vi "AOTF Messenger.vi"(0 "AOTF Notifier Name":string, 2 "AOTF Action":T1, 5 "Wavelength (nm)":string, 7 "Power (%)":dbl, 9 "Line On/Off":bool, 11 "Beam Blank":bool) -> (4 "AOTF Notifier Name (Dup)":string, 6 "Wavelength (nm) Out":string, 8 "Power (%) Out":dbl, 10 "Line On/Off Out":bool, 13 "Wavelengths (nm)":string[](array[string]), 15 "Beam Blank Out":bool)   [LabVIEW 2016]
uses:
  AOTF Controls/AOTF Actions.ctl
  AOTF Controls/AOTF Notifier Element.ctl
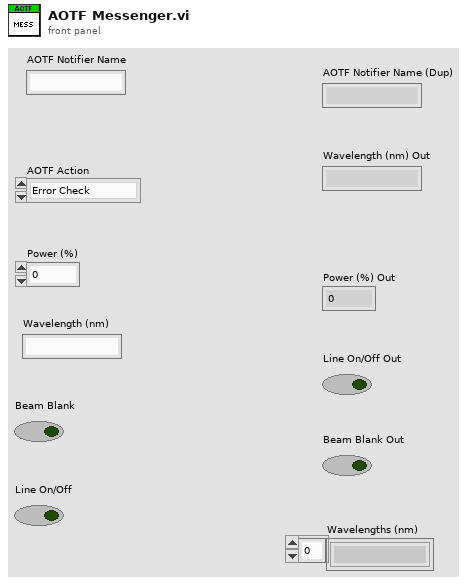
[diagram p1: front panel]
types:
  T1 = typedef "AOTF Actions.ctl" = enum16{"Error Check", "Blank", "Line On/Off", "Set Power", "Status", "Quit"}
  T2 = typedef "AOTF Notifier Element.ctl" = cluster{"AOTF Action":T1, "Laser Line":string, "Power (%)":dbl, "Beam Blank On/Off":bool, "Line On/Off":bool, "Error":errorcluster, "Wavelengths (nm)":string[]}
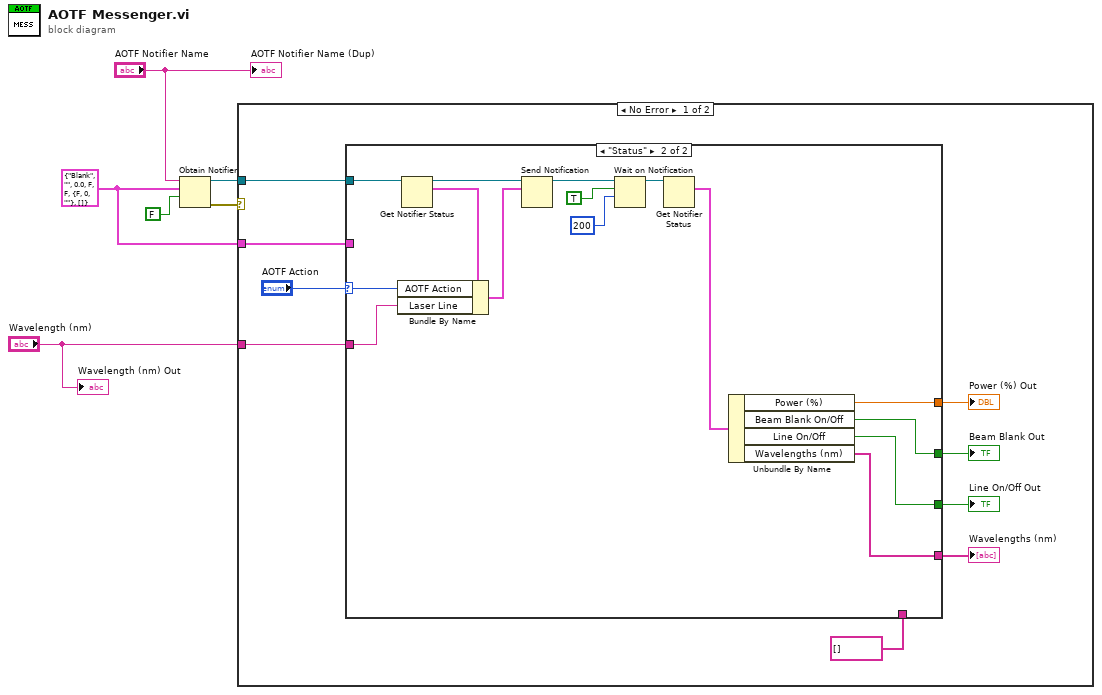
[diagram p0: block diagram]
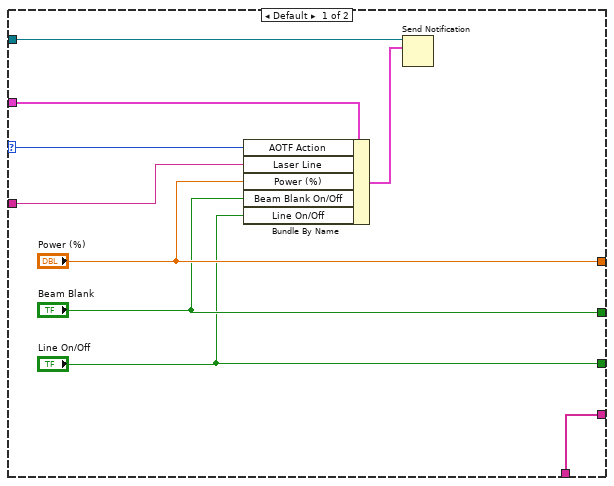
[diagram p2: hidden frame]
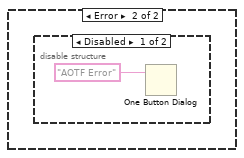
[diagram p3: hidden frame]
diagram:
  w2 = T2 {"AOTF Action"=enum."Blank", "Laser Line"="", "Power (%)"=0.0, "Beam Blank On/Off"=FALSE, "Line On/Off"=FALSE, "Error"={"status"=FALSE, "code"=0, "source"=""}, "Wavelengths (nm)"=[]} ("AOTFQueueCtrl")
  n1 = Obtain Notifier(name (unnamed)="AOTF Notifier Name", notification data type=w2, create if not found? (T)=FALSE) -> (notifier out=w4:refnum<notifier>, error out=w3:errorcluster)  [unwired: 1 in, 1 out]
  n2 = case shown="No Error" w3 {
    tunnel: w4 -> [w15 _]
    tunnel: w2 -> [w14 _]
    tunnel: "Wavelength (nm)" -> [w13 _]
    frame No Error {
      n3 = case shown="\"Status\"" "AOTF Action" {
        selector: "AOTF Action" -> [w20 w32]
        tunnel: w15 -> [w24 w35]
        tunnel: w14 -> [w23 _]
        tunnel: w13 -> [w21 w26]
        tunnel: ["Power (%)" w38] -> w9
        tunnel: ["Beam Blank" w36] -> w10
        tunnel: ["Line On/Off" w37] -> w11
        tunnel: [w16 w25] -> w8
        tunnel: string[] [] ("Wavelengths (nm)") -> [w16 _]
        frame Default {
          n4 = Bundle By Name(cluster=w23, "AOTF Action"=w20, "Laser Line"=w21, "Power (%)"="Power (%)", "Beam Blank On/Off"="Beam Blank", "Line On/Off"="Line On/Off") -> (w22:T2)
          n5 = Send Notification(notification=w22, notifier=w24) -> ()  [unwired: 1 in, 2 out]
        }
        frame "Status" {
          n6 = Get Notifier Status(notifier=w35) -> (notifier out=w34:refnum<notifier>, current notification=w33:T2)  [unwired: 1 in, 3 out]
          n7 = Bundle By Name(cluster=w33, "AOTF Action"=w32, "Laser Line"=w26) -> (w31:T2)
          n8 = Send Notification(notification=w31, notifier=w34) -> (notifier out=w30:refnum<notifier>)  [unwired: 1 in, 1 out]
          n9 = Wait on Notification(notifier=w30, ignore previous (F)=TRUE, timeout in ms (-1)=200) -> (notifier out=w27:refnum<notifier>)  [unwired: 1 in, 3 out]
          n10 = Get Notifier Status(notifier=w27) -> (current notification=w39:T2)  [unwired: 1 in, 4 out]
          n11 = Unbundle By Name(w39) -> ("Power (%)"=w38:dbl, "Beam Blank On/Off"=w36:bool, "Line On/Off"=w37:bool, "Wavelengths (nm)"=w25:string[])
        }
      }
      "Line On/Off Out" <- w11
      "Beam Blank Out" <- w10
      "Power (%) Out" <- w9
      "Wavelengths (nm)" <- w8
    }
    frame Error {
      n12 = disable-structure shown="Disabled" {
        frame Disabled {
          n13 = One Button Dialog(message="AOTF Error") -> ()  [unwired: 1 in, 1 out]
        }
        frame Enabled {
        }
      }
    }
  }
  "AOTF Notifier Name (Dup)" <- "AOTF Notifier Name"
  "Wavelength (nm) Out" <- "Wavelength (nm)"
